vi "Write Param.vi"(8 "error in (no error)":errorcluster, 10 "Param":dbl[][](array[numeric]), 11 "Param in":T1) -> (0 "error out":errorcluster, 3 "Param out":T1)   [LabVIEW 2019]
uses:
  Ctl/Param.ctl
  Inputs.lvlib
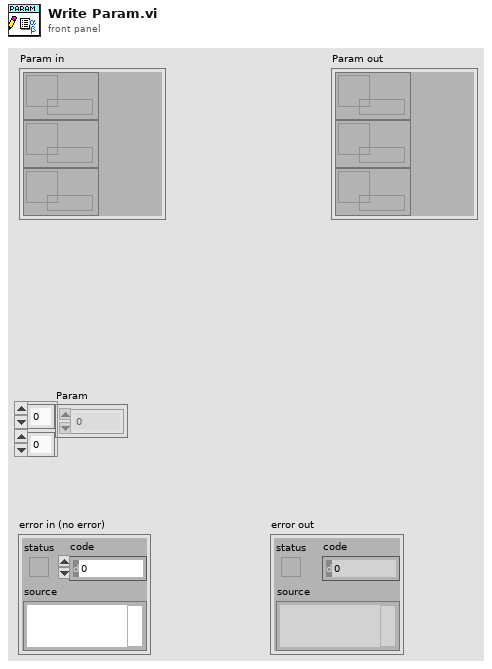
[diagram p1: front panel]
types:
  T1 = typedef "Inputs.lvlib/Param.ctl" = cluster{"modified":refnum<data-value>, "PAR":refnum<data-value>, "PARNames":refnum<data-value>}
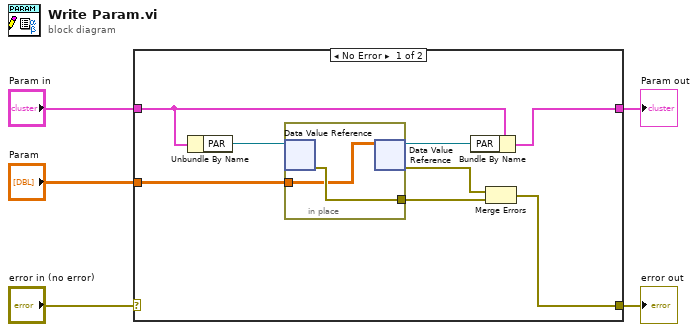
[diagram p0: block diagram]
diagram:
  n1 = case shown="No Error" "error in (no error)" {
    selector: "error in (no error)" -> [_ w17]
    tunnel: [w6 w17] -> w4
    tunnel: [w9 w16] -> w2
    tunnel: "Param in" -> [w11 w16]
    tunnel: "Param" -> [w12 _]
    frame No Error {
      n2 = Unbundle By Name(w11) -> ("PAR"=w13:refnum<data-value>)
      n3 = in-place {
        in-place-border: w12 -> [w14]
        in-place-border: [w15] -> w7
        n4 = in-place-dvr #1(w13) -> (w15:errorcluster)  [unwired: 1 out]
        n5 = in-place-dvr #1(w14) -> (w10:refnum<data-value>, w8:errorcluster)
      }
      n6 = Bundle By Name(cluster=w11, "PAR"=w10) -> (w9:T1)
      n7 = Merge Errors(w8, w7) -> (w6:errorcluster)
    }
    frame Error {
    }
  }
  "error out" <- w4
  "Param out" <- w2
